vi "FTW-Connector-SendPoisonPill.vi"(0 "FTW Actor Connector":refnum<data-value>, 5 "Timeout":i32=1000 format="%dmsec", 11 "error in":errorcluster) -> (4 "FTW Actor Connector out":refnum<data-value>, 6 "Shutting Down?":bool, 8 "Roundtrip Time":dbl format="%.4psec", 15 "error out":errorcluster)   [LabVIEW 2014]
uses:
  socket/connector/core/FTW-Connector-Core-Type.ctl
  error/FTW-ERR-ThrowError.vi
  lib/FTW-KernelFilepath.vi
  error/FTW-ERR-CallChain.vi
  string/FTW-STR-ReplaceWhitespace.vi
  json/core/FTW-JSON-Core-EncodingFlags.vi
  reflection/FTW-Reflection-Type.vi
  codegen/xnode/json/fetch/FTW-JSON-Core-GetFlattenedValue.vi
  codegen/xnode/FTW-JSON-Fetch.xnode
panel:
  # "Inputs"
  # "Outputs"
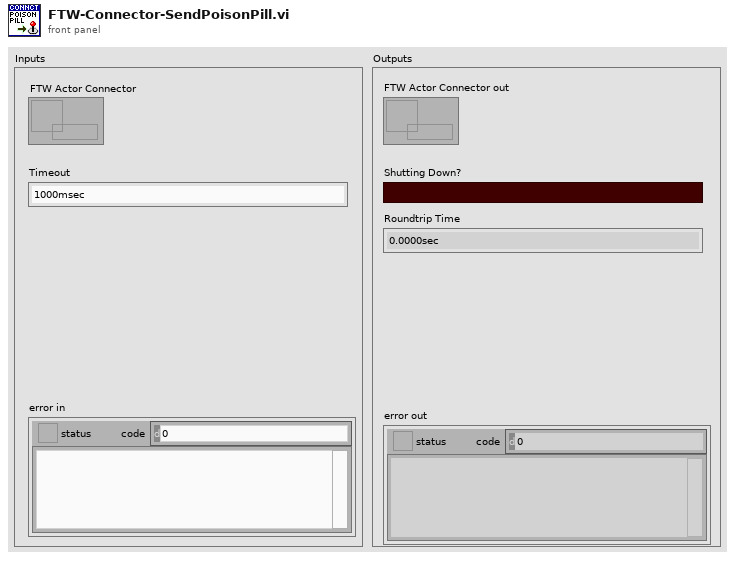
[diagram p1: front panel]
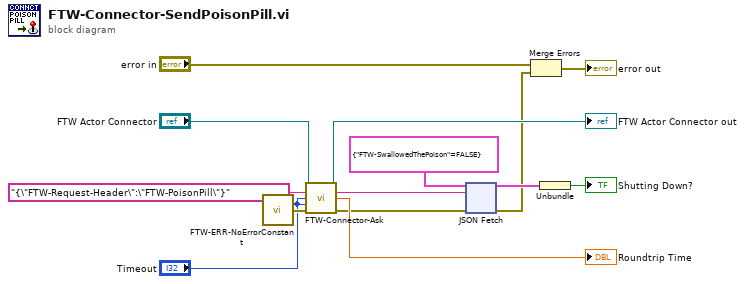
[diagram p0: block diagram]
diagram:
  n1 = call "FTW-ERR-NoErrorConstant.vi"() -> ("no error"=w10:errorcluster)
  n2 = call "FTW-Connector-Ask.vi"("FTW Actor Connector"="FTW Actor Connector", "Request"="{\"FTW-Request-Header\":\"FTW-PoisonPill\"}", "Receive Timeout"="Timeout", "Send Timeout"="Timeout", "error in"=w10) -> ("FTW Actor Connector out"=→"FTW Actor Connector out":refnum<data-value>, "Response"=w6:string, "Roundtrip Time"=→"Roundtrip Time":dbl, "error out"=w5:errorcluster)  [unwired: 7 in]
  n3 = xnode "JSON Fetch"("Type and Defaults"=cluster{"FTW-SwallowedThePoison":bool} {"FTW-SwallowedThePoison"=FALSE}, "JSON String"=w6, "error in"=w5) -> ("Values"=w4:cluster{"FTW-SwallowedThePoison":bool}, "error out"=w3:errorcluster)  [unwired: 1 in]
  n4 = Merge Errors("error in", w3) -> (→"error out":errorcluster)
  n5 = Unbundle(w4) -> ("FTW-SwallowedThePoison"=→"Shutting Down?":bool)
